vi "HW initialize at start.vi"(8 "error in (no error)":errorcluster, 11 "mmWave instr in":refnum<class "mmWave instrument.lvclass">) -> (0 "error out":errorcluster, 3 "mmW instr out":refnum<class "mmWave instrument.lvclass">)   [LabVIEW 2019, in "HW Control.lvlib"]
uses:
  HW Control.lvlib
  SubVIs/mmWave instrument_class/mmWave instrument.lvclass
  SubVIs/Shared/System GV.vi
  SubVIs/Shared/Shared.lvlib
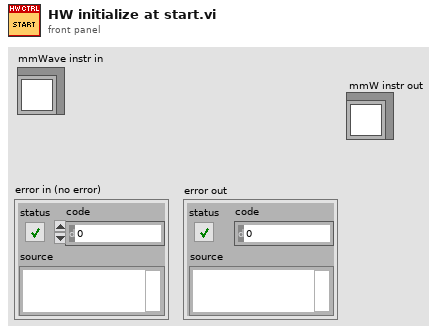
[diagram p1: front panel]
types:
  T1 = cluster{"Boolean Round":bool, "code":i32, "source":string}
  T2 = typedef "TX trigger config.ctl" = cluster{"delay":dbl, "trig source":T3, "PXI src":i32, "export":T4, "PXI dest":i32}
  T3 = typedef "FPGA Utility.lvlib/FPGA driver trigger source.ctl" = enum16{"Use Tclk", "PXI_Trig", "Aurora RX trig"}
  T4 = typedef "FPGA Utility.lvlib/FPGA driver trigger destination.ctl" = enum16{"None", "Source trig", "Synced trig", "Delayed sync"}
  T5 = typedef "mmWave HW Control.lvlib/LO export.ctl" = cluster{"TX LO1 export":bool, "TX LO1 export level":dbl, "RX LO1 export":bool, "RX LO1 export level":dbl, "LO2 export":bool, "LO2 export level":dbl}
  T6 = typedef "mmWave HW Control.lvlib/LO sources.ctl" = cluster{"RX/LO1 src":string, "TX/LO1 src":string, "LO2 src":string}
  T7 = typedef "mmWave instrument.lvclass/Sync mode.ctl" = enum16{"Slave", "Master"}
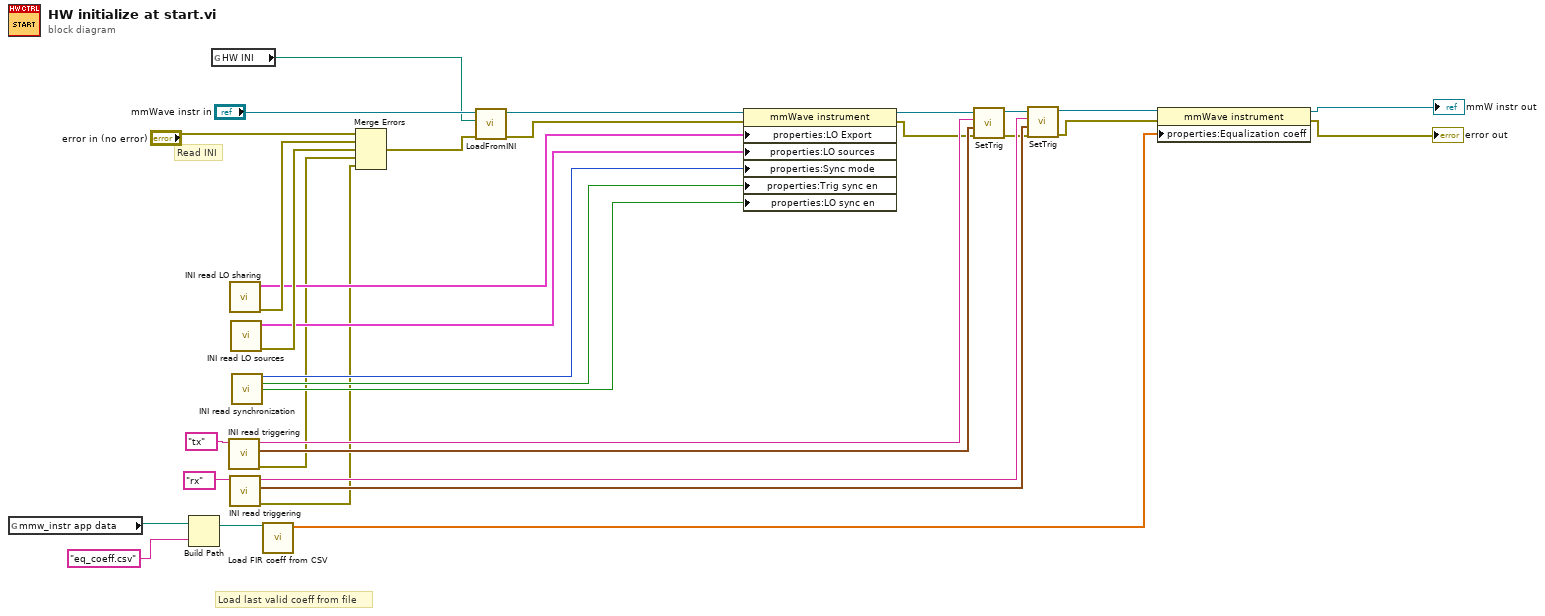
[diagram p0: block diagram]
diagram:
  # "Load last valid coeff from file"
  # "Read INI"
  n1 = global read "System GV.vi" "mmw_instr app data"() -> (w16:path)
  n2 = Build Path(base path=w16, name or relative path="eq_coeff.csv") -> (appended path=w4:path)
  n3 = global read "System GV.vi" "HW INI"() -> (w11:path)
  n4 = call "INI read triggering.vi"("Port"="tx") -> ("error out"=w2:T1, "Trig opt"=w31:T2, "Port out"=w30:string)  [unwired: 8 in]
  n5 = call "INI read LO sharing.vi"() -> ("error out"=w22:T1, "data"=w20:T5)  [unwired: 10 in]
  n6 = call "INI read triggering.vi"("Port"="rx") -> ("error out"=w1:T1, "Trig opt"=w33:T2, "Port out"=w32:string)  [unwired: 8 in]
  n7 = call "INI read LO sources.vi"() -> ("error out"=w23:T1, "data"=w21:T6)  [unwired: 10 in]
  n8 = call "INI read synchronization.vi"() -> ("Sync mode"=w7:T7, "Trig sync en"=w6:bool, "LO sync en"=w5:bool)  [unwired: 12 in, 1 out]
  n9 = call "Load FIR coeff from CSV.vi"("Path"=w4) -> ("1D Array"=w15:cdb[])  [unwired: 8 in, 2 out]
  n10 = Merge Errors("error in (no error)", w22, w23, w2, w1) -> (w10:errorcluster)
  n11 = call-dynamic "LoadFromINI.vi"("error in (no error)"=w10, "path"=w11, "reference in"="mmWave instr in") -> ("error out"=w8:errorcluster, "reference out"=w9:refnum<class "mmWave instrument.lvclass">)  [unwired: 7 in]
  n12 = property class="mmWave instrument"(reference=w9, error in=w8, "properties:LO Export"=w20, "properties:LO sources"=w21, "properties:Sync mode"=w7, "properties:Trig sync en"=w6, "properties:LO sync en"=w5) -> (reference out=w25:refnum<class "mmWave instrument.lvclass">, error out=w24:errorcluster)
  n13 = call-dynamic "SetTrig.vi"("error in (no error)"=w24, "TX trigger options"=w31, "Port"=w30, "reference in"=w25) -> ("error out"=w29:errorcluster, "reference out"=w28:refnum<class "mmWave instrument.lvclass">)  [unwired: 6 in]
  n14 = call-dynamic "SetTrig.vi"("error in (no error)"=w29, "TX trigger options"=w33, "Port"=w32, "reference in"=w28) -> ("error out"=w26:errorcluster, "reference out"=w27:refnum<class "mmWave instrument.lvclass">)  [unwired: 6 in]
  n15 = property class="mmWave instrument"(reference=w27, error in=w26, "properties:Equalization coeff"=w15) -> (reference out=→"mmW instr out":refnum<class "mmWave instrument.lvclass">, error out=→"error out":errorcluster)
